vi "WPI_RobotDriveOpen6MotorWithSPARK.vi"(0 "Rear Left Motor":T1=enum."Invalid", 1 "Rear Right Motor":T1=enum."Invalid", 2 "Front Left Motor":T1=enum."Invalid", 3 "Front Right Motor":T1=enum."Invalid", 4 "Middle Left Motor":T1=enum."Invalid", 5 "error in (no error)":errorcluster, 7 "Middle Right Motor":T1=enum."Invalid", 8 "Rear Left Motor Inverted":bool, 9 "Front Left Motor Inverted":bool, 10 "Rear Right Motor Inverted":bool, 11 "Front Right Motor Inverted":bool, 12 "Middle Left Motor Inverted":bool, 13 "Middle Right Motor Inverted":bool) -> (14 "RobotDriveDevRef":T2={"DevStatus"={"status"=FALSE, "code"=0, "source"=""}, "Motors[]"=[], "Square Inputs"=FALSE, "Max Output"=1.0}, 19 "error out":errorcluster)   [LabVIEW 2018]
doc: "Opens a reference to the robot drive for a four-motor robot using Rev Robotics SPARK motor controllers.\n\nThis software is licensed. Open the labview\\readme\\WPI Robotics Library Open Source License.txt file for more information."
uses:
  <vilib>/Rock Robotics/SystemInterfaces/DIO/FPGA_DIOPWMChannel.ctl
  <vilib>/Rock Robotics/WPI/RobotDrive/WPI_RobotDriveDevRef.ctl
  <vilib>/Rock Robotics/WPI/MotorControl/WPI_MotorControlDeviceRef.ctl
  <vilib>/Rock Robotics/WPI/MotorControl/WPI_MotorControlType.ctl
  <vilib>/Rock Robotics/WPI/PWM/WPI_PWMDeadband.ctl
  <vilib>/Rock Robotics/SystemInterfaces/DIO/FPGA_DIOChannel.ctl
  <vilib>/Rock Robotics/WPI/SafetyOutput/WPI_SafetyOutputConfigMenu.ctl
  <vilib>/Rock Robotics/WPI/MotorControl/WPI_MotorControlOpen SPARK.vi
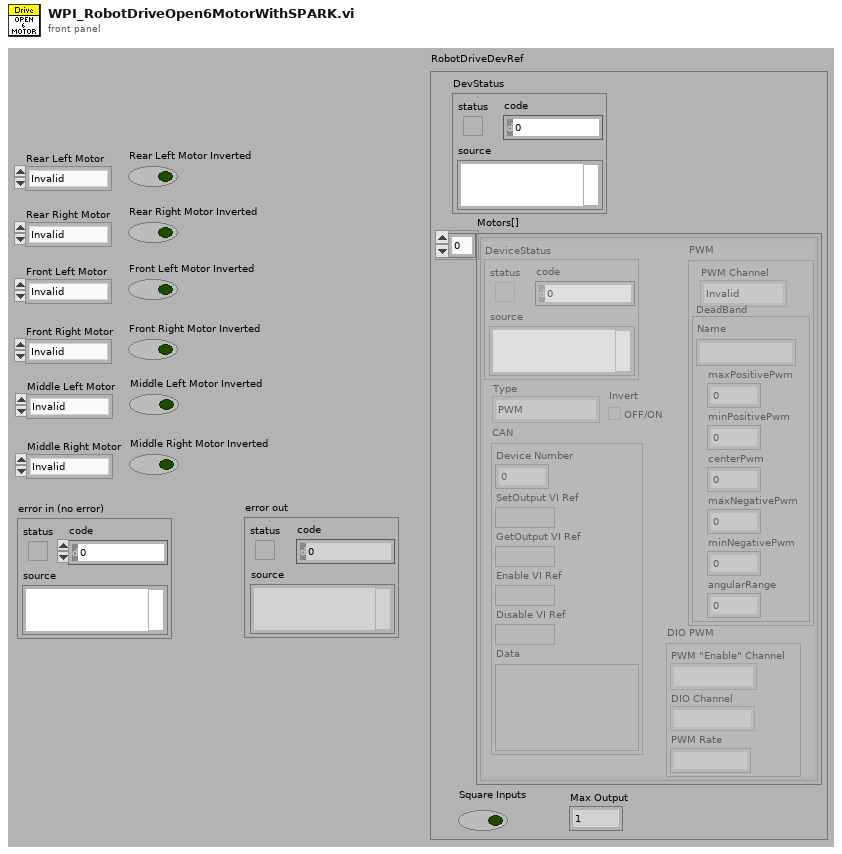
[diagram p1: front panel]
types:
  T1 = typedef "FPGA_DIOPWMChannel.ctl" = enum8{"PWM 0", "PWM 1", "PWM 2", "PWM 3", "PWM 4", "PWM 5", "PWM 6", "PWM 7", "PWM 8", "PWM 9", "PWM MXP 0", "PWM MXP 1", "PWM MXP 2", "PWM MXP 3", "PWM MXP 4", "PWM MXP 5", "PWM MXP 6", "PWM MXP 7", "PWM MXP 8", "PWM MXP 9", "Invalid"}
  T2 = typedef "WPI_RobotDriveDevRef.ctl" = cluster{"DevStatus":errorcluster, "Motors[]":T3[], "Square Inputs":bool, "Max Output":dbl}
  T3 = typedef "WPI_MotorControlDeviceRef.ctl" = cluster{"DeviceStatus":errorcluster, "Type":T4, "PWM":cluster{"PWM Channel":T1, "DeadBand":T5}, "CAN":cluster{"Device Number":u8, "SetOutput VI Ref":variant, "GetOutput VI Ref":variant, "Enable VI Ref":variant, "Disable VI Ref":variant, "Data":variant}, "Invert":bool, "DIO PWM":cluster{"PWM \"Enable\" Channel":T1, "DIOChannel":T6, "PWM Rate":dbl}}
  T4 = typedef "WPI_MotorControlType.ctl" = enum16{"PWM", "CAN", "DIO PWM"}
  T5 = typedef "WPI_PWMDeadband.ctl" = cluster{"Name":string, "maxPositivePwm":i32, "minPositivePwm":i32, "centerPwm":i32, "maxNegativePwm":i32, "minNegativePwm":i32, "angularRange":u16}
  T6 = typedef "FPGA_DIOChannel.ctl" = enum8{"DIO 0", "DIO 1", "DIO 2", "DIO 3", "DIO 4", "DIO 5", "DIO 6", "DIO 7", "DIO 8", "DIO 9", "DIO MXP 0", "DIO MXP 1", "DIO MXP 2", "DIO MXP 3", "DIO MXP 4", "DIO MXP 5", "DIO MXP 6", "DIO MXP 7", "DIO MXP 8", "DIO MXP 9", "DIO MXP 10", "DIO MXP 11", "DIO MXP 12", "DIO MXP 13", "DIO MXP 14", "DIO MXP 15", "SPI Port CS1", "SPI Port CS2", "SPI Port CS3", "SPI Port MISO", "SPI Port MOSI", "Invalid"}
  T7 = typedef "WPI_SafetyOutputConfigMenu.ctl" = enum16{"Enable", "Disable"}
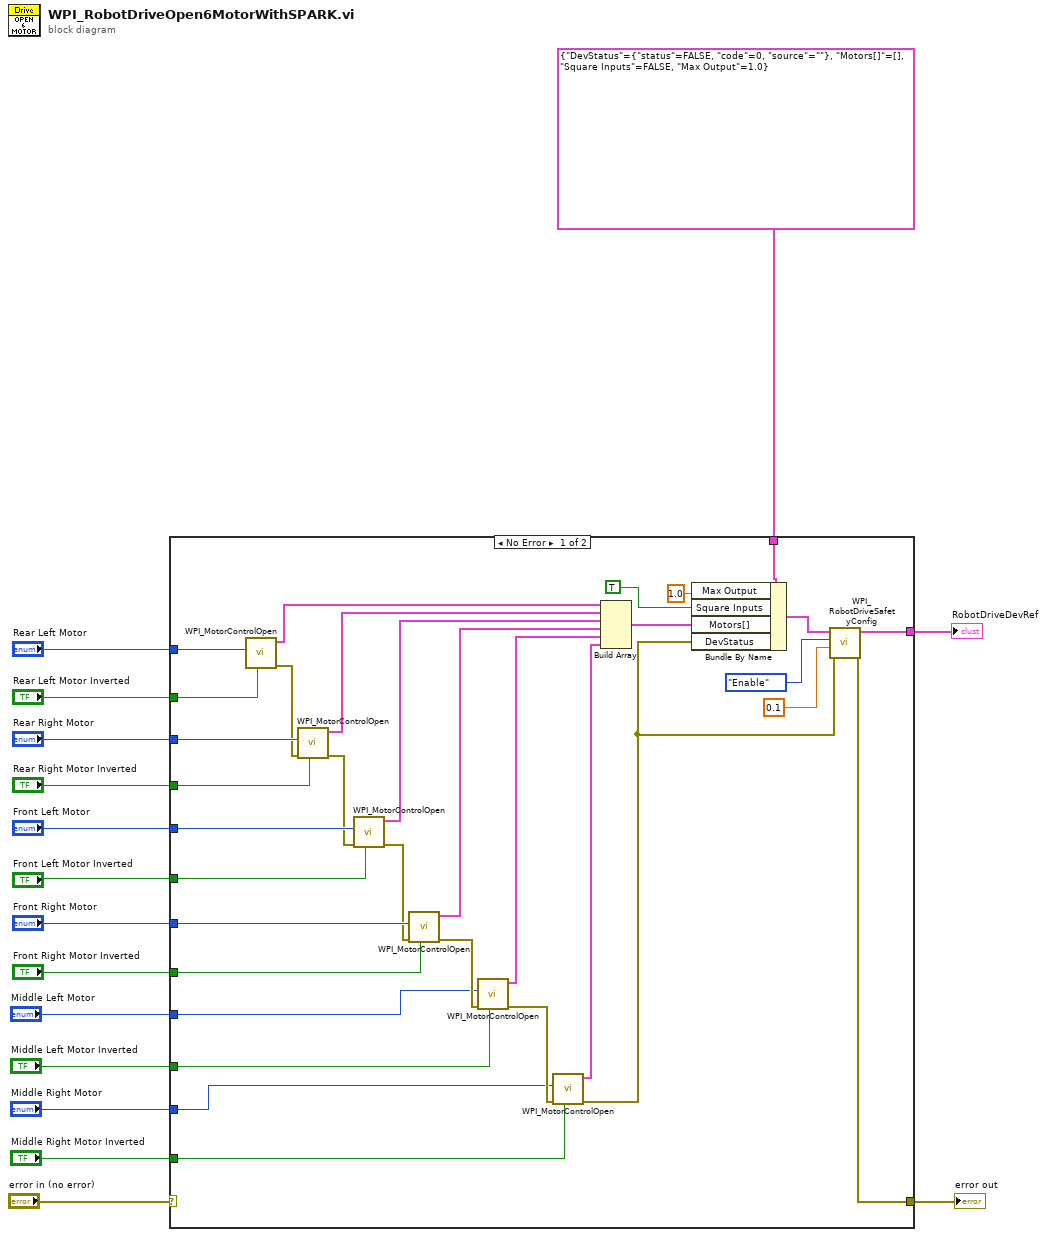
[diagram p0: block diagram]
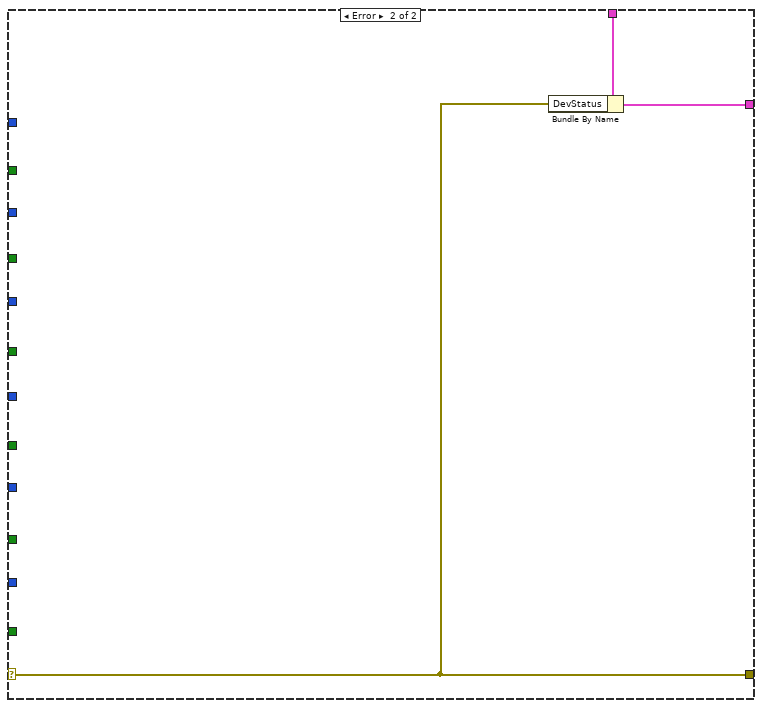
[diagram p2: hidden frame]
diagram:
  n1 = case shown="No Error" "error in (no error)" {
    selector: "error in (no error)" -> [_ w50]
    tunnel: [w28 w51] -> w16
    tunnel: T2 {"DevStatus"={"status"=FALSE, "code"=0, "source"=""}, "Motors[]"=[], "Square Inputs"=FALSE, "Max Output"=1.0} ("RobotDriveDevRef") -> [w49 w52]
    tunnel: "Rear Left Motor" -> [w47 _]
    tunnel: "Front Right Motor" -> [w44 _]
    tunnel: "Front Left Motor" -> [w45 _]
    tunnel: "Rear Right Motor" -> [w46 _]
    tunnel: "Rear Left Motor Inverted" -> [w35 _]
    tunnel: "Rear Right Motor Inverted" -> [w34 _]
    tunnel: "Front Right Motor Inverted" -> [w32 _]
    tunnel: "Front Left Motor Inverted" -> [w33 _]
    tunnel: [w29 w50] -> w5
    tunnel: "Middle Left Motor" -> [w22 _]
    tunnel: "Middle Left Motor Inverted" -> [w21 _]
    tunnel: "Middle Right Motor Inverted" -> [w20 _]
    tunnel: "Middle Right Motor" -> [w19 _]
    frame No Error {
      n2 = call-poly <vilib>:"WPI_MotorControlOpen.vi"("Invert"=w35, "PWM Channel"=w47) -> ("error out"=w37:errorcluster, "MotorControlDeviceRef"=w43:T3)  [unwired: 2 in, 6 out]
      n3 = call-poly <vilib>:"WPI_MotorControlOpen.vi"("Invert"=w34, "error in (no error)"=w37, "PWM Channel"=w46) -> ("error out"=w38:errorcluster, "MotorControlDeviceRef"=w42:T3)  [unwired: 1 in, 6 out]
      n4 = call-poly <vilib>:"WPI_MotorControlOpen.vi"("Invert"=w33, "error in (no error)"=w38, "PWM Channel"=w45) -> ("error out"=w39:errorcluster, "MotorControlDeviceRef"=w41:T3)  [unwired: 1 in, 6 out]
      n5 = call-poly <vilib>:"WPI_MotorControlOpen.vi"("Invert"=w32, "error in (no error)"=w39, "PWM Channel"=w44) -> ("error out"=w23:errorcluster, "MotorControlDeviceRef"=w40:T3)  [unwired: 1 in, 6 out]
      n6 = call-poly <vilib>:"WPI_MotorControlOpen.vi"("Invert"=w21, "error in (no error)"=w23, "PWM Channel"=w22) -> ("error out"=w25:errorcluster, "MotorControlDeviceRef"=w18:T3)  [unwired: 1 in, 6 out]
      n7 = call-poly <vilib>:"WPI_MotorControlOpen.vi"("Invert"=w20, "error in (no error)"=w25, "PWM Channel"=w19) -> ("error out"=w24:errorcluster, "MotorControlDeviceRef"=w17:T3)  [unwired: 1 in, 6 out]
      n8 = Build Array(w43, w42, w41, w40, w18, w17) -> (w36:T3[])
      n9 = Bundle By Name(cluster=w49, "Max Output"=1.0, "Square Inputs"=TRUE ("DestroyPWM?"), "Motors[]"=w36, "DevStatus"=w24) -> (w30:T2)
      n10 = call <vilib>:"WPI_RobotDriveSafetyConfig.vi"("error in (no error)"=w24, "timeout (s)"=0.1, "mode"=WPI_SafetyOutputConfigMenu."Enable", "RobotDriveDevRef"=w30) -> ("error out"=w29:errorcluster, "RobotDriveDevRef"=w28:T2)  [unwired: 6 out]
    }
    frame Error {
      n11 = Bundle By Name(cluster=w52, "DevStatus"=w50) -> (w51:T2)
    }
  }
  "RobotDriveDevRef" <- w16
  "error out" <- w5
